vi "Monitoreo.vi"() -> ()   [LabVIEW 2020]
uses:
  <vilib>/Instr/_visa.llb/VISA Configure Serial Port (Instr).vi
panel:
  in  "Escribir":bool
  in  "stop":bool
  out "Mensaje":string
  in  "Write":string
  out "Lectura random":string
  in  "Leer":bool
  in  "VISA resource name":refnum<visa-resource-name>
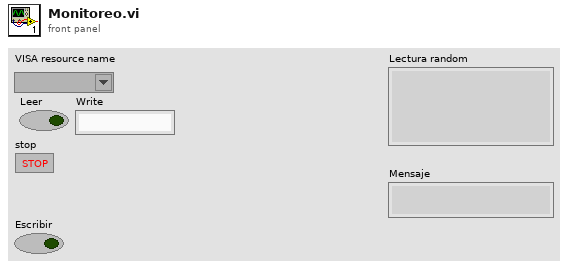
[diagram p1: front panel]
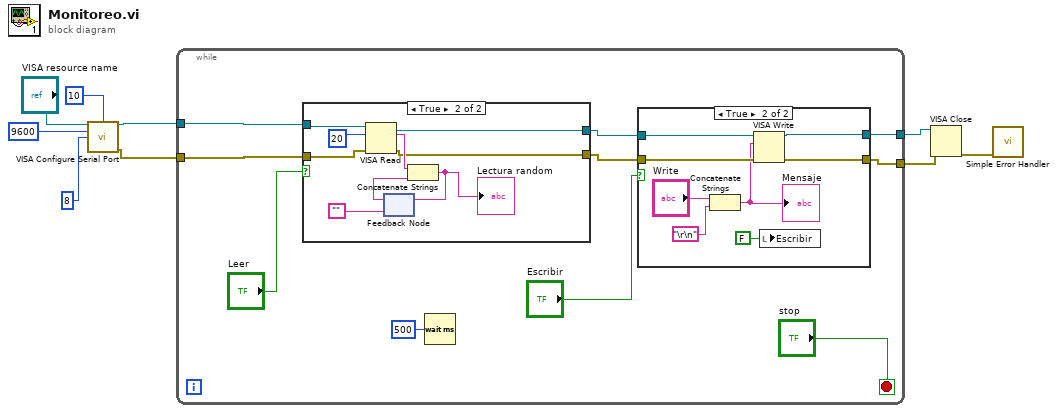
[diagram p0: block diagram]
diagram:
  n1 = call-poly "VISA Configure Serial Port"("VISA resource name"="VISA resource name", "termination char\n(0xA = '\\n' = LF)"=u8 10 ("termination char\n(0xA = '\\n' = LF)"), "baud rate (9600)"=u32 9600, "data bits (8)"=u16 8) -> ("VISA resource name out"=w5:refnum<visa-resource-name>, "error out"=w4:errorcluster)  [unwired: 10 in]
  n2 = while {
    tunnel: w5 -> [w19]
    tunnel: w4 -> [w17]
    tunnel: [w11] -> w2
    tunnel: [w10] -> w1
    stop <- "stop" stop-if-true
    n3 = case shown="True" "Leer" {
      tunnel: w19 -> [w31 w40]
      tunnel: w17 -> [w30 w39]
      tunnel: [w31 w34] -> w13
      tunnel: [w30 w33] -> w12
      frame False {
      }
      frame True {
        n4 = VISA Read(VISA resource name=w40, byte count=u32 20, error in (no error)=w39) -> (VISA resource name out=w34:refnum<visa-resource-name>, read buffer=w37:string, error out=w33:errorcluster)  [unwired: 1 out]
        n5 = feedback #1("") -> (w35:string)
        n6 = Concatenate Strings(w37, w35) -> (w36:string)
        "Lectura random" <- w36
        n7 = feedback-in #1(w36) -> ()
      }
    }
    n8 = Wait (ms)(milliseconds to wait=u32 500) -> ()  [unwired: 1 out]
    n9 = case shown="True" "Escribir" {
      tunnel: w13 -> [w21 w29]
      tunnel: w12 -> [w20 w28]
      tunnel: [w21 w25] -> w11
      tunnel: [w20 w24] -> w10
      frame False {
      }
      frame True {
        n10 = Concatenate Strings("Write", "\r\n") -> (w26:string)
        "Mensaje" <- w26
        n11 = VISA Write(VISA resource name=w29, write buffer=w26, error in (no error)=w28) -> (VISA resource name out=w25:refnum<visa-resource-name>, error out=w24:errorcluster)  [unwired: 1 out]
        n12 = local write "Escribir"(FALSE ("Escribir")) -> ()
      }
    }
  }
  n13 = VISA Close(VISA resource name=w2, error in (no error)=w1) -> (error out=w3:errorcluster)
  n14 = call <vilib>:"Simple Error Handler.vi"("error in (no error)"=w3) -> ()  [unwired: 4 in, 5 out]
